vi "ReadAndInvokeMatlabEvents.vi"(10 "ExperimentID":string, 11 "User Event in":refnum<user-event>) -> ()   [LabVIEW 2017]
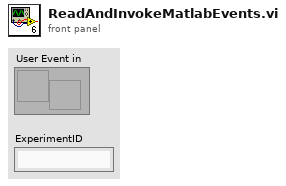
[diagram p1: front panel]
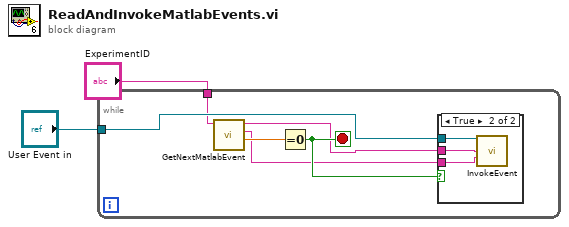
[diagram p0: block diagram]
diagram:
  n1 = while {
    tunnel: "User Event in" -> [w4]
    tunnel: "ExperimentID" -> [w3]
    stop <- w7 stop-if-true
    n2 = call "GetNextMatlabEvent.vi"("ExperimentID"=w3) -> ("Numeric"=w8:dbl, "String 2"=w6:string, "String"=w5:string)  [unwired: 8 in]
    n3 = Equal To 0?(x=w8) -> (x = 0?=w7:bool)
    n4 = case shown="True" w7 {
      tunnel: w6 -> [_ w11]
      tunnel: w5 -> [_ w10]
      tunnel: w4 -> [_ w9]
      frame False {
      }
      frame True {
        n5 = call "InvokeEvent.vi"("Event Stream In"=w9, "name"=w10, "Data"=w11) -> ()  [unwired: 11 in, 2 out]
      }
    }
  }
